vi "Open.vi"(8 "error in":errorcluster, 9 "parameters":variant, 10 "file path":path, 11 "SequenceRepo In":refnum<class "SequenceRepo.lvclass">) -> (0 "error out":errorcluster, 2 "invalid?":bool, 3 "SequenceRepo out":refnum<class "SequenceRepo.lvclass">)   [LabVIEW 2015, in "SequenceRepo.lvclass"]
doc: "Here we are specifying to read the configuration from a gXML file. And version managementCopyright 2017 National Instruments Corporation\n\nLicensed under the Apache License, Version 2.0 (the \"License\"); you may not use this file except in compliance with the License. You may obtain a copy of the License at http://www.apache.org/licenses/LICENSE-2.0\nUnless required by applicable law or agreed to in writing, software distributed under the License is distributed on an \"AS IS\" BASIS, WITHOUT WARRANTIES OR CONDITIONS OF ANY KIND, either express or implied. See the License for the specific language governing permissions and limitations under the License."
uses:
  SequenceRepo.lvclass
  SequenceRepo.lvclass/SequenceRepo.ctl
  <vilib>/Utility/file.llb/Read Delimited Spreadsheet (string).vi
  Prototype/classes/Sequence/Config/Sequence Config.lvclass
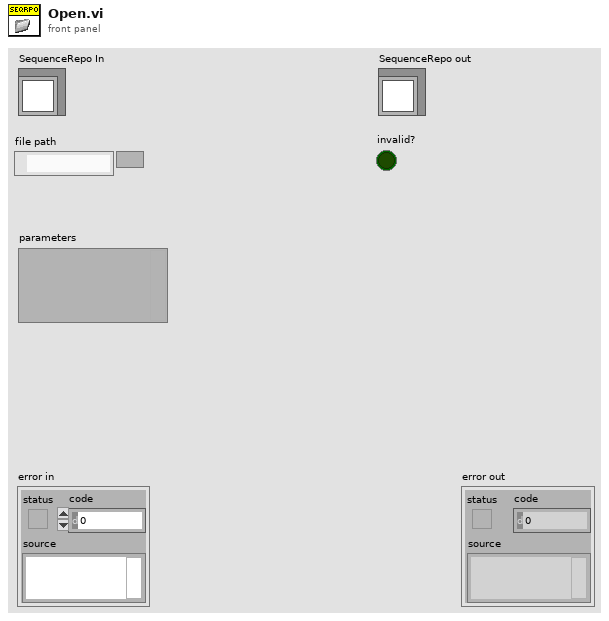
[diagram p1: front panel]
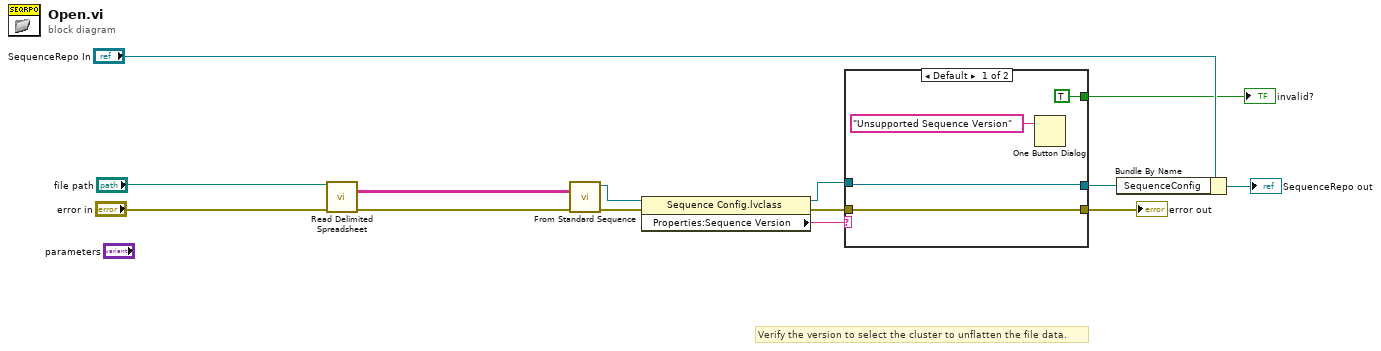
[diagram p0: block diagram]
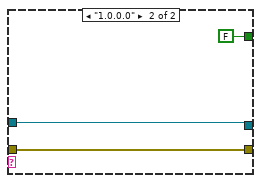
[diagram p2: hidden frame]
diagram:
  # "Verify the version to select the cluster to unflatten the file data."
  n1 = call-poly <vilib>:"Read Delimited Spreadsheet.vi"("file path (dialog if empty)"="file path", "error in (no error)"="error in") -> ("all rows"=w1:string[][], "error out"=w3:errorcluster)  [unwired: 8 in, 4 out]
  n2 = call "From Standard Sequence.vi"("error in (no error)"=w3, "Standard Sequence"=w1) -> ("error out"=w8:errorcluster, "Sequence Config.lvclass"=w6:refnum<class "Sequence Config.lvclass">)  [unwired: 8 in]
  n3 = property class="Sequence Config.lvclass"(reference=w6, error in=w8) -> (reference out=w4:refnum<class "Sequence Config.lvclass">, error out=w7:errorcluster, "Properties:Sequence Version"=w5:string)
  n4 = case shown="Default" w5 {
    tunnel: [w15 w20] -> w11
    tunnel: [w18 w19] -> w9
    tunnel: w7 -> [w18 w19]
    tunnel: [TRUE FALSE] -> w10
    tunnel: w4 -> [w15 w20]
    frame Default {
      n5 = One Button Dialog(message="Unsupported Sequence Version") -> ()  [unwired: 1 in, 1 out]
    }
    frame "1.0.0.0" {
    }
  }
  "error out" <- w9
  "invalid?" <- w10
  n6 = Bundle By Name(cluster="SequenceRepo In", "SequenceConfig"=w11) -> (→"SequenceRepo out":refnum<class "SequenceRepo.lvclass">)
